vi "Add_Part_of_Track(After_101)_Two_Problems-1.vi"(4 "[IN] Index in subtrack":i32, 5 "[IN] Minimal Sub\ntrack Length":i32, 6 "[IN] Subtrack":T2, 7 "[IN] Indexes for Jumps":i32[](array[numeric]), 8 "error IN":errorcluster, 9 "[IN] Count of variants":i32, 10 "[IN] Subtracks":T1(array[cluster]), 11 "[IN] Still connected\ntracks in group":T3) -> (0 "error OUT":errorcluster, 1 "[OUT] Count of variants":i32, 2 "[OUT] Subtracks":T1(array[cluster]))   [LabVIEW 2013]
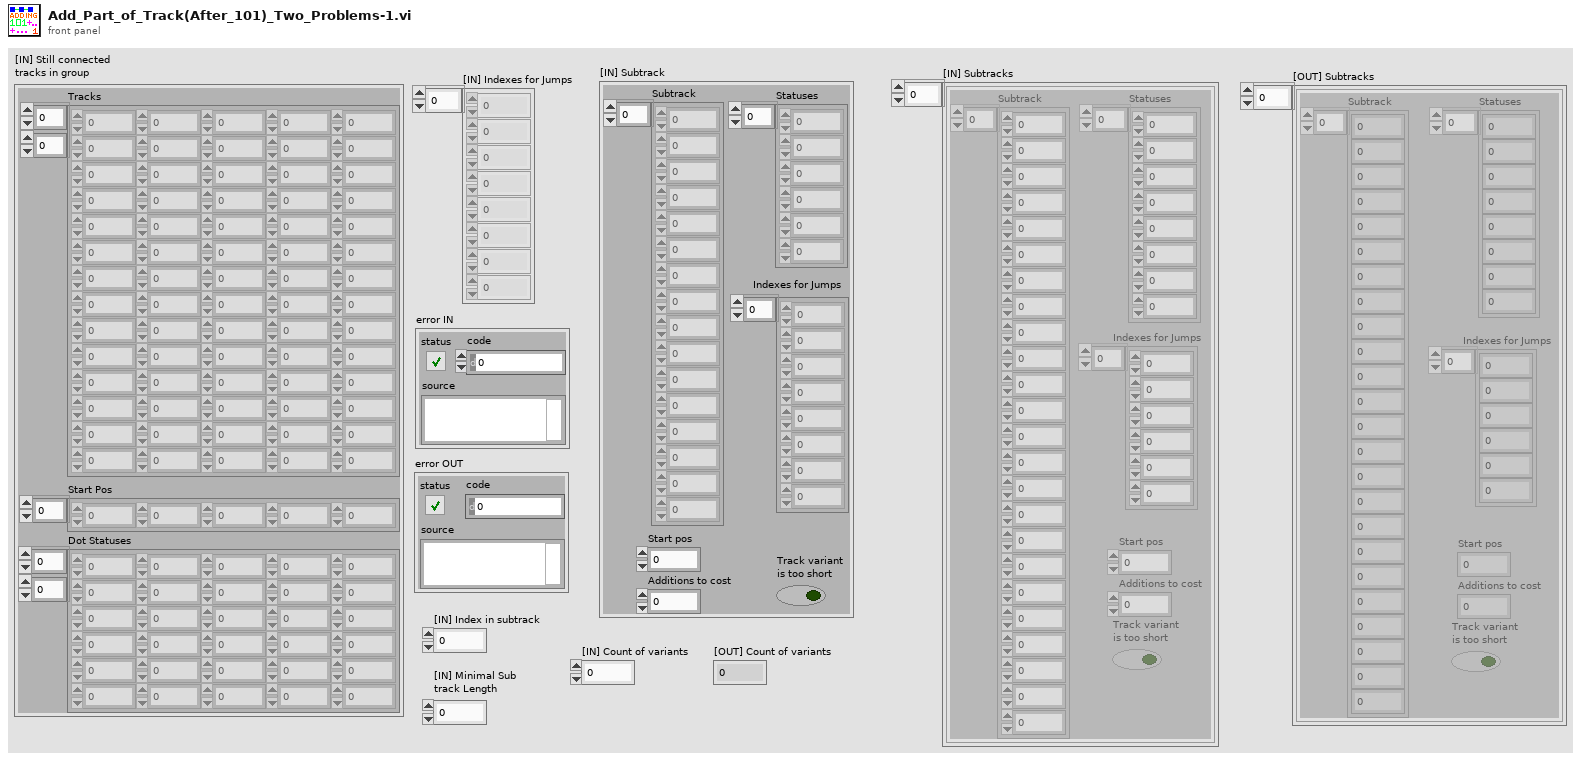
[diagram p1: front panel]
types:
  T1 = cluster{"Subtrack":dbl[], "Statuses":i16[], "Start pos":i32, "Additions to cost":i32, "Track variant \nis too short":bool, "Indexes for Jumps":i32[]}[]
  T2 = cluster{"Subtrack":dbl[], "Statuses":i16[], "Start pos":i32, "Additions to cost":i32, "Track variant \nis too short":bool, "Indexes for Jumps":i32[]}
  T3 = cluster{"Tracks":dbl[][], "Start Pos":i32[], "Dot Statuses":i16[][]}
  T4 = cluster{"Subtrack":dbl[], "Statuses":i16[], "Start pos":i32, "Additions to cost":i8, "Track variant \nis too short":bool, "Indexes for Jumps":i32[]}
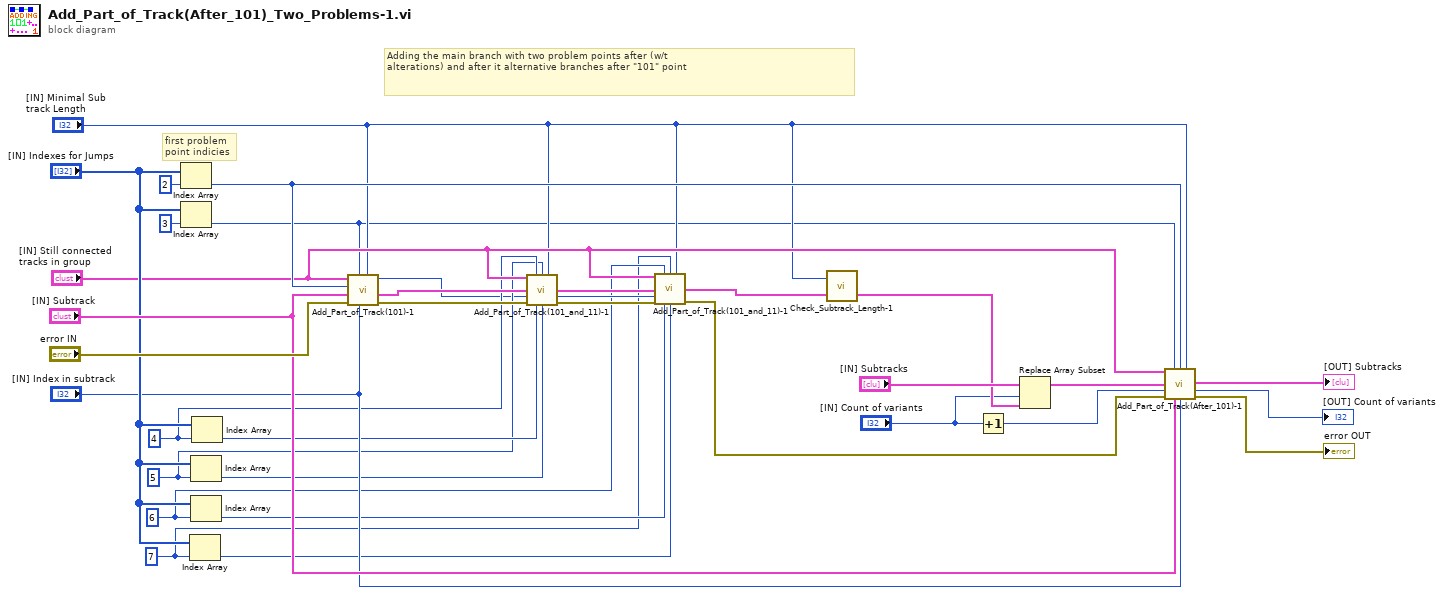
[diagram p0: block diagram]
diagram:
  w2 = 7 ("index")
  w3 = 6 ("index")
  w6 = 5 ("index")
  w7 = 4 ("index")
  # "first problem \npoint indicies"
  # "Adding the main branch with two problem points after (w/t \nalterations) and after it alternative branches after \"101\" point"
  n1 = Index Array(array="[IN] Indexes for Jumps", index=2) -> (element=w24:i32)
  n2 = Index Array(array="[IN] Indexes for Jumps", index=3) -> (element=w10:i32)
  n3 = Index Array(array="[IN] Indexes for Jumps", index=w2) -> (element=w4:i32)
  n4 = Index Array(array="[IN] Indexes for Jumps", index=w6) -> (element=w8:i32)
  n5 = Index Array(array="[IN] Indexes for Jumps", index=w3) -> (element=w5:i32)
  n6 = Index Array(array="[IN] Indexes for Jumps", index=w7) -> (element=w9:i32)
  n7 = call "Add_Part_of_Track(101)-1.vi"("[IN] Minimal Sub\ntrack Length"="[IN] Minimal Sub\ntrack Length", "[IN] Index in subtrack"="[IN] Index in subtrack", "[IN] # of subtrack conta\nining problem point"=w10, "error IN"="error IN", "[IN] Subtrack"="[IN] Subtrack", "[IN] Index of problem\npoint inside subtrack"=w24, "[IN] Still connected\ntracks in group"="[IN] Still connected\ntracks in group") -> ("error OUT"=w31:errorcluster, "[OUT] Subtrack"=w17:T2, "[OUT] Last point in subtrack"=w1:i32)  [unwired: 2 in]
  n8 = call "Add_Part_of_Track(101_and_11)-1.vi"("[IN] Still connected\ntracks in group"="[IN] Still connected\ntracks in group", "[IN] i for Probl\nem  Point Index"=w7, "[IN] i for # of Track \nwith Problem Point"=w6, "[IN] Minimal Sub\ntrack Length"="[IN] Minimal Sub\ntrack Length", "[IN] Subtrack"=w17, "[IN] Index in subtrack"=w1, "error IN"=w31, "[IN] Index of problem\npoint inside subtrack"=w9, "[IN] # of subtrack conta\nining problem point"=w8) -> ("[OUT] Subtrack"=w15:T2, "[OUT] Last point in subtrack"=w14:i32, "error OUT"=w19:errorcluster)  [unwired: 4 in]
  n9 = call "Add_Part_of_Track(101_and_11)-1.vi"("[IN] Still connected\ntracks in group"="[IN] Still connected\ntracks in group", "[IN] i for Probl\nem  Point Index"=w3, "[IN] i for # of Track \nwith Problem Point"=w2, "[IN] Minimal Sub\ntrack Length"="[IN] Minimal Sub\ntrack Length", "[IN] Subtrack"=w15, "[IN] Index in subtrack"=w14, "error IN"=w19, "[IN] Index of problem\npoint inside subtrack"=w5, "[IN] # of subtrack conta\nining problem point"=w4) -> ("[OUT] Subtrack"=w11:T2, "error OUT"=w18:errorcluster)  [unwired: 4 in, 1 out]
  n10 = call "Check_Subtrack_Length-1.vi"("[IN] Subtrack"=w11, "[IN] Minimal Sub\ntrack Length"="[IN] Minimal Sub\ntrack Length") -> ("[OUT] Subtrack"=w29:T4)  [unwired: 1 in]
  n11 = Increment(x="[IN] Count of variants") -> (x+1=w26:i32)
  n12 = Replace Array Subset(array="[IN] Subtracks", new element=w29, index="[IN] Count of variants") -> (w27:T1)
  n13 = call "Add_Part_of_Track(After_101)-1.vi"("[IN] Still connected\ntracks in group"="[IN] Still connected\ntracks in group", "[IN] # of subtrack conta\nining problem point"=w10, "[IN] Index of problem\npoint inside subtrack"=w24, "[IN] Minimal Sub\ntrack Length"="[IN] Minimal Sub\ntrack Length", "[IN] Subtracks"=w27, "[IN] Count of variants"=w26, "error IN"=w18, "[IN] Subtrack"="[IN] Subtrack", "[IN] Index in subtrack"="[IN] Index in subtrack") -> ("[OUT] Subtracks"=→"[OUT] Subtracks":T1, "[OUT] Count of variants"=→"[OUT] Count of variants":i32, "error OUT"=→"error OUT":errorcluster)  [unwired: 4 in]
